vi "node_info.vi"(1 "Length":i32[](array[numeric]), 2 "Type":i32, 3 "Name":string) -> (0 "Info":string)   [LabVIEW 2011]
panel:
  # "0: numeric\n1: string"
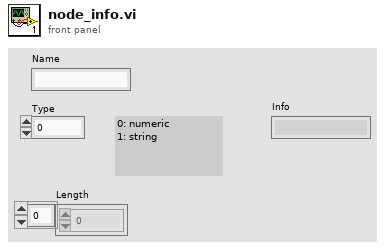
[diagram p1: front panel]
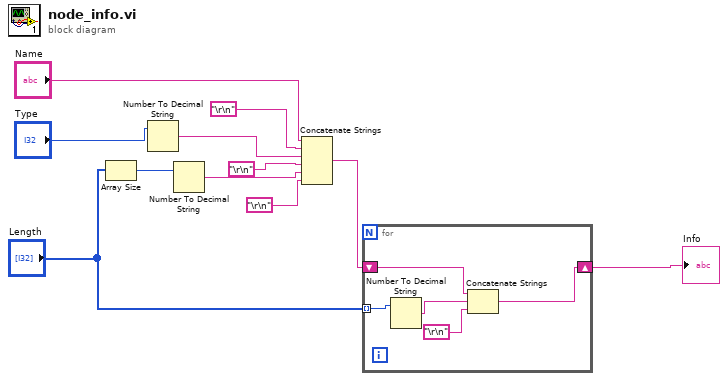
[diagram p0: block diagram]
diagram:
  n1 = Array Size(array="Length") -> (size(s)=w9:i32)
  n2 = Number To Decimal String(number="Type") -> (decimal integer string=w1:string)  [unwired: 1 in]
  n3 = Number To Decimal String(number=w9) -> (decimal integer string=w4:string)  [unwired: 1 in]
  n4 = Concatenate Strings("Name", "\r\n", w1, "\r\n", w4, "\r\n") -> (w6:string)
  n5 = for {
    tunnel: "Length" -> [w15] mode=indexing
    shift-right: [w12] -> w5
    shift-left: w6 -> [w13]
    n6 = Number To Decimal String(number=w15) -> (decimal integer string=w16:string)  [unwired: 1 in]
    n7 = Concatenate Strings(w13, w16, "\r\n") -> (w12:string)
  }
  "Info" <- w5
